vi "Call Set Build Exclusions.vi"(8 "error in (no error)":errorcluster, 11 "Build Spec Info in":T1) -> (0 "error out":errorcluster)   [LabVIEW 2010]
uses:
  Types/Job Type.ctl
  Types/Task Info.ctl
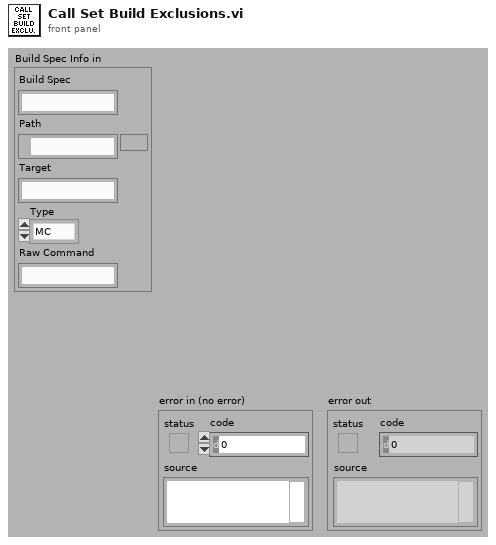
[diagram p1: front panel]
types:
  T1 = typedef "Task Info.ctl" = cluster{"Build Spec":string, "Path":path, "Target":string, "Type":T2, "Raw Command":string}
  T2 = typedef "Job Type.ctl" = enum16{"MC", "NOP", "VI", "Build", "VIP", "VIPB", "VIA"}
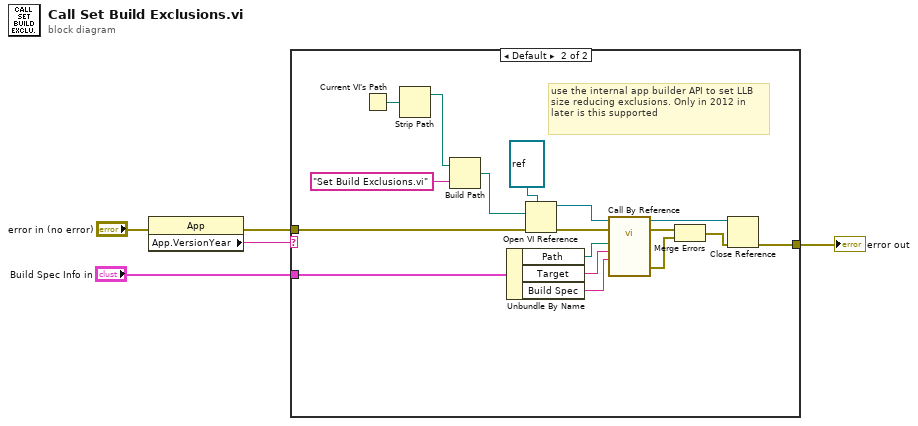
[diagram p0: block diagram]
diagram:
  n1 = property class="App"(error in="error in (no error)") -> (error out=w2:errorcluster, "App.VersionYear"=w1:string)  [unwired: 1 in, 1 out]
  n2 = case shown="Default" w1 {
    tunnel: "Build Spec Info in" -> [_ w11]
    tunnel: [w6 w8] -> w3
    tunnel: w2 -> [w6 w7]
    frame "2010", "2011" {
    }
    frame Default {
      # "use the internal app builder API to set LLB size reducing exclusions. Only in 2012 in later is this supported"
      n3 = Current VI's Path() -> (path=w21:path)
      n4 = Strip Path(path=w21) -> (stripped path=w20:path)  [unwired: 1 out]
      n5 = Build Path(base path=w20, name or relative path="Set Build Exclusions.vi") -> (appended path=w19:path)
      n6 = Unbundle By Name(w11) -> ("Path"=w14:path, "Target"=w13:string, "Build Spec"=w12:string)
      n7 = Open VI Reference(type specifier VI Refnum (for type only)=refnum<vi> refnum, vi path=w19, error in (no error)=w7) -> (vi reference=w18:refnum<vi>, error out=w17:errorcluster)  [unwired: 3 in]
      n8 = call-by-ref "?"(reference=w18, error in=w17, "Build specification name"=w12, "target name"=w13, "Source project"=w14) -> (reference out=w9:refnum<vi>, error out=w16:errorcluster, 0:"error out"=w15:errorcluster)  [unwired: 8 in]
      n9 = Merge Errors(w16, w15) -> (w10:errorcluster)
      n10 = Close Reference(reference=w9, error in (no error)=w10) -> (error out=w8:errorcluster)
    }
  }
  "error out" <- w3
